vi "Configure VIP Uninstall.vi"(8 "error in (no error)":errorcluster, 10 "JSON string":string) -> (0 "error out":errorcluster, 3 "VIP Install Out":refnum<class "VIPM Update.lvclass">)   [LabVIEW 2014, in "VIPM Update.lvclass"]
uses:
  VIPM Update.lvclass
  Shared/Controls/VIPM Update - STYP.ctl
  VIPM Update.lvclass/VIPM Update.ctl
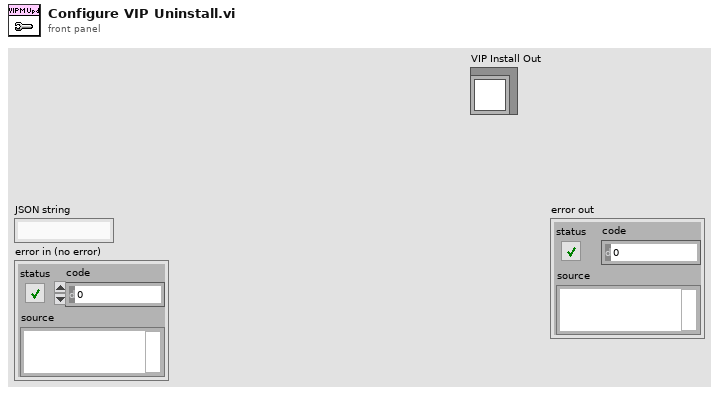
[diagram p1: front panel]
types:
  T1 = typedef "VIPM Update - STYP.ctl" = cluster{"LabVIEW Version":string}
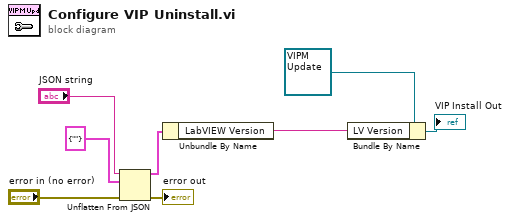
[diagram p0: block diagram]
diagram:
  n1 = Unflatten From JSON(JSON string="JSON string", type and defaults=T1 {"LabVIEW Version"=""} ("VIP Publish"), error in (no error)="error in (no error)") -> (value=w4:T1, error out=→"error out":errorcluster)  [unwired: 4 in]
  n2 = Unbundle By Name(w4) -> ("LabVIEW Version"=w2:string)
  n3 = Bundle By Name(cluster=refnum<class "VIPM Update.lvclass"> refnum ("VIPB Build out"), "LV Version"=w2) -> (→"VIP Install Out":refnum<class "VIPM Update.lvclass">)
